vi "Set Photon Counting Threshold.vi"(10 "max":i32, 11 "min":i32) -> (3 "function return":u32)   [LabVIEW 2018, in "AndorSDK.lvlib"]
doc: "EXPNETTYPE unsigned int WINAPI SetPhotonCountingThreshold(long min, long max);"
uses:
  AndorSDK.lvlib
  ATMCD32D.dll
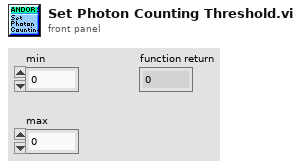
[diagram p1: front panel]
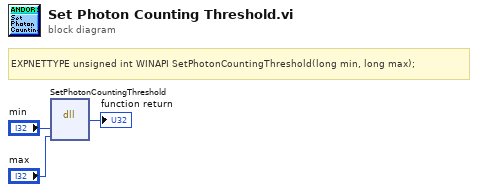
[diagram p0: block diagram]
diagram:
  # "EXPNETTYPE unsigned int WINAPI SetPhotonCountingThreshold(long min, long max);"
  n1 = dll-call lib="PTH2babs E\nPersönliches02 - Arbeit03-HiwijobsLabviewCodelibANDOR\tAndor SDK\nATMCD32D.*" fn="SetPhotonCountingThreshold"("min"="min", "max"="max") -> (→"function return":u32)  [unwired: 5 in, 2 out]
